vi "add photostim filename to protocol notes.vi"(10 "stim power":dbl, 11 "rec start/end (T is start)":bool) -> (3 "protocol.notes out":string)   [LabVIEW 2012]
doc: "SciScan 1.0 151216"
uses:
  GFG/GFGstringGet.vi
  GFG/GFGfpRefGet.vi
  GFG/GFG library.lvlib
panel:
  in  "file path":string
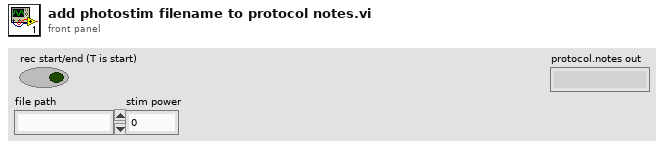
[diagram p1: front panel]
types:
  T1 = cluster{"WaveformChartRef":refnum<vi>, "DigitalRef":refnum<vi>, "ArrayRef":refnum<vi>, "TabControlRef":refnum<vi>, "EnumRef":refnum<vi>, "RingRef":refnum<vi>, "BooleanRef":refnum<vi>, "KnobRef":refnum<vi>, "SlideRef":refnum<vi>, "PathRef":refnum<vi>, "StringRef":refnum<vi>, "ComboBox":refnum<vi>, "WaveformGraphRef":refnum<vi>}
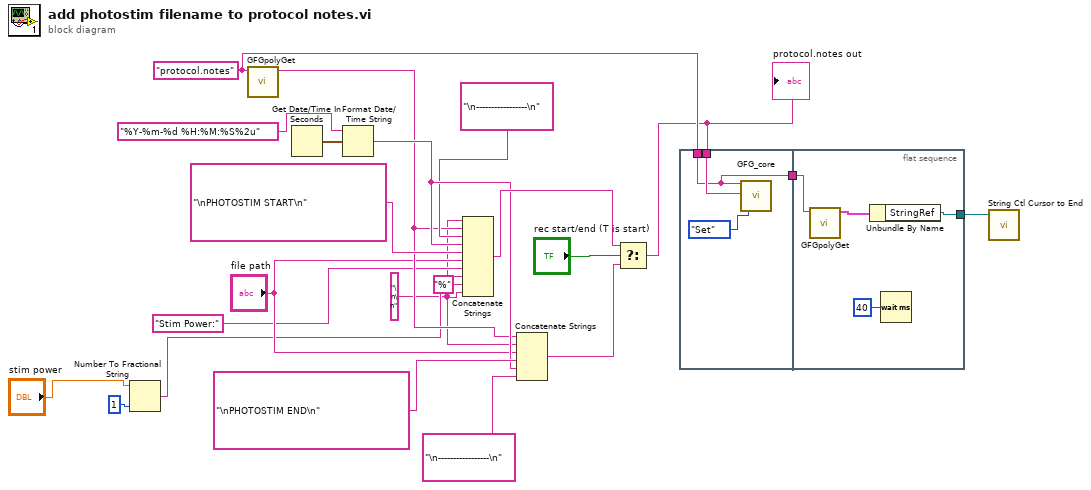
[diagram p0: block diagram]
diagram:
  w3 = "\n\n" ("string")
  w21 = "protocol.notes" ("Variable Name in")
  n1 = Number To Fractional String(number="stim power", precision (6)=i16 1 ("width (-)")) -> (F-format string=w4:string)  [unwired: 2 in]
  n2 = call-poly "GFGpolyGet.vi"("Variable Name in"=w21) -> ("String"=w8:string)  [unwired: 9 in, 1 out]
  n3 = Get Date/Time In Seconds() -> (seconds since 1Jan1904=w12:timestamp)
  n4 = Format Date/Time String(time format string (%c)="%Y-%m-%d %H:%M:%S%2u", seconds (now)=w12) -> (date/time string=w10:string)  [unwired: 1 in]
  n5 = Concatenate Strings(w3, w8, "\n-----------------\n" ("string"), w10, "\nPHOTOSTIM START\n" ("string"), "file path", "Stim Power:" ("string"), w4, "%" ("string"), w3) -> (w19:string)
  n6 = Concatenate Strings(w8, w3, "file path", "\nPHOTOSTIM END\n" ("string"), w10, "\n-----------------\n" ("string")) -> (w17:string)
  n7 = Select(t=w19, s="rec start/end (T is start)", f=w17) -> (s? t:f=w18:string)
  "protocol.notes out" <- w18
  n8 = flat-sequence {
    tunnel: w21 -> [w23]
    tunnel: w18 -> [w24]
    tunnel: [w23] -> w15
    tunnel: w15 -> [w29]
    tunnel: [w27] -> w14
    frame #0 {
      n9 = call "GFG_core.vi"("Variable Name in"=w23, "Variant in"=w24, "Action"=enum16{"Init", "Set", "Get"}."Set") -> ()  [unwired: 10 in, 7 out]
    }
    frame #1 {
      n10 = call-poly "GFGpolyGet.vi"("Variable Name in"=w29) -> ("output cluster"=w28:T1)  [unwired: 9 in, 1 out]
      n11 = Unbundle By Name(w28) -> ("StringRef"=w27:refnum<vi>)
      n12 = Wait (ms)(milliseconds to wait=u32 40) -> ()  [unwired: 1 out]
    }
  }
  n13 = call "String Ctl Cursor to End.vi"("String Reference in"=w14) -> ()  [unwired: 10 in, 1 out]
